vi "vision mapping.vi"(10 "GIC Input":T2={"     Use ?\nOff       On"=[FALSE, TRUE, FALSE, TRUE], "Mode:"=FALSE, "Extra Port"="", "Hokuyo Port"="COM7", "Tx Prop  Port"="COM6", "Compass Port"="", "GPS Port"="", "Num of WPs"=0, "WP Lats and Longs"={"WP Lats"=[], "WP Longs"=[]}, "Obst Lats and Longs"={"Obst Lats"=[], "Obst Longs"=[]}, "Parameters"=[], "GPS Data"=[], "Compass"=0.0, "LMS Vector"=[], "Vision Vector"=[], "Direction Cmd"=0.0, "Speed Cmd"=0.0, "WP Vector"=[], "WP Number"=0, "Extra"=0, "SW Map"=[], "Path Cluster"={"Path x node"=[], "Path y node"=[]}, "Sim Course"=[]} {"Obst Lats and Longs"."Obst Longs" format="%#_8g"; "Obst Lats and Longs"."Obst Lats" format="%#_8g"}, 11 "From vision processing":dbl[][](array[numeric])=array492x658[323736 elements]) -> (2 "GIC Output":T1={"     Use ?\nOff       On"=[FALSE, TRUE, FALSE, TRUE], "Mode:"=FALSE, "Extra Port"="", "Hokuyo Port"="COM7", "Tx Prop Port"="COM6", "Compass Port"="", "GPS Port"="", "Num of WPs"=0, "WP Lats and Longs"={"WP Lats"=[], "WP Longs"=[]}, "Obst Lats and Longs"={"Obst Lats"=[], "Obst Longs"=[]}, "Parameters"=[], "GPS Data"=[], "Compass"=0.0, "LMS Vector"=[], "Vision Vector"=[], "Direction Cmd"=0.0, "Speed Cmd"=0.0, "WP Vector"=[], "WP Number"=0, "Extra"=0, "SW Map"=[], "Path Cluster"={"Path x node"=[], "Path y node"=[]}, "Sim Course"=[]} {"Obst Lats and Longs"."Obst Longs" format="%#_8g"; "Obst Lats and Longs"."Obst Lats" format="%#_8g"})   [LabVIEW 2014]
panel:
  out "image out":T3(plugin-control)
  out "Local Map":picture
  out "tes7":dbl
  out "tes6":dbl
  out "tes5":dbl
  out "tes4":dbl
  out "tes3":dbl
  out "tes2":dbl
  out "xn2":dbl
  out "yn1":dbl
  out "xn1":dbl
  out "th":dbl
  out "ppm":dbl
  out "yp":dbl
  out "xp":dbl
  out "SwMap out":dbl[][](array[numeric])
  # "Vision Mapping"
  # "Input:"
  # "Output"
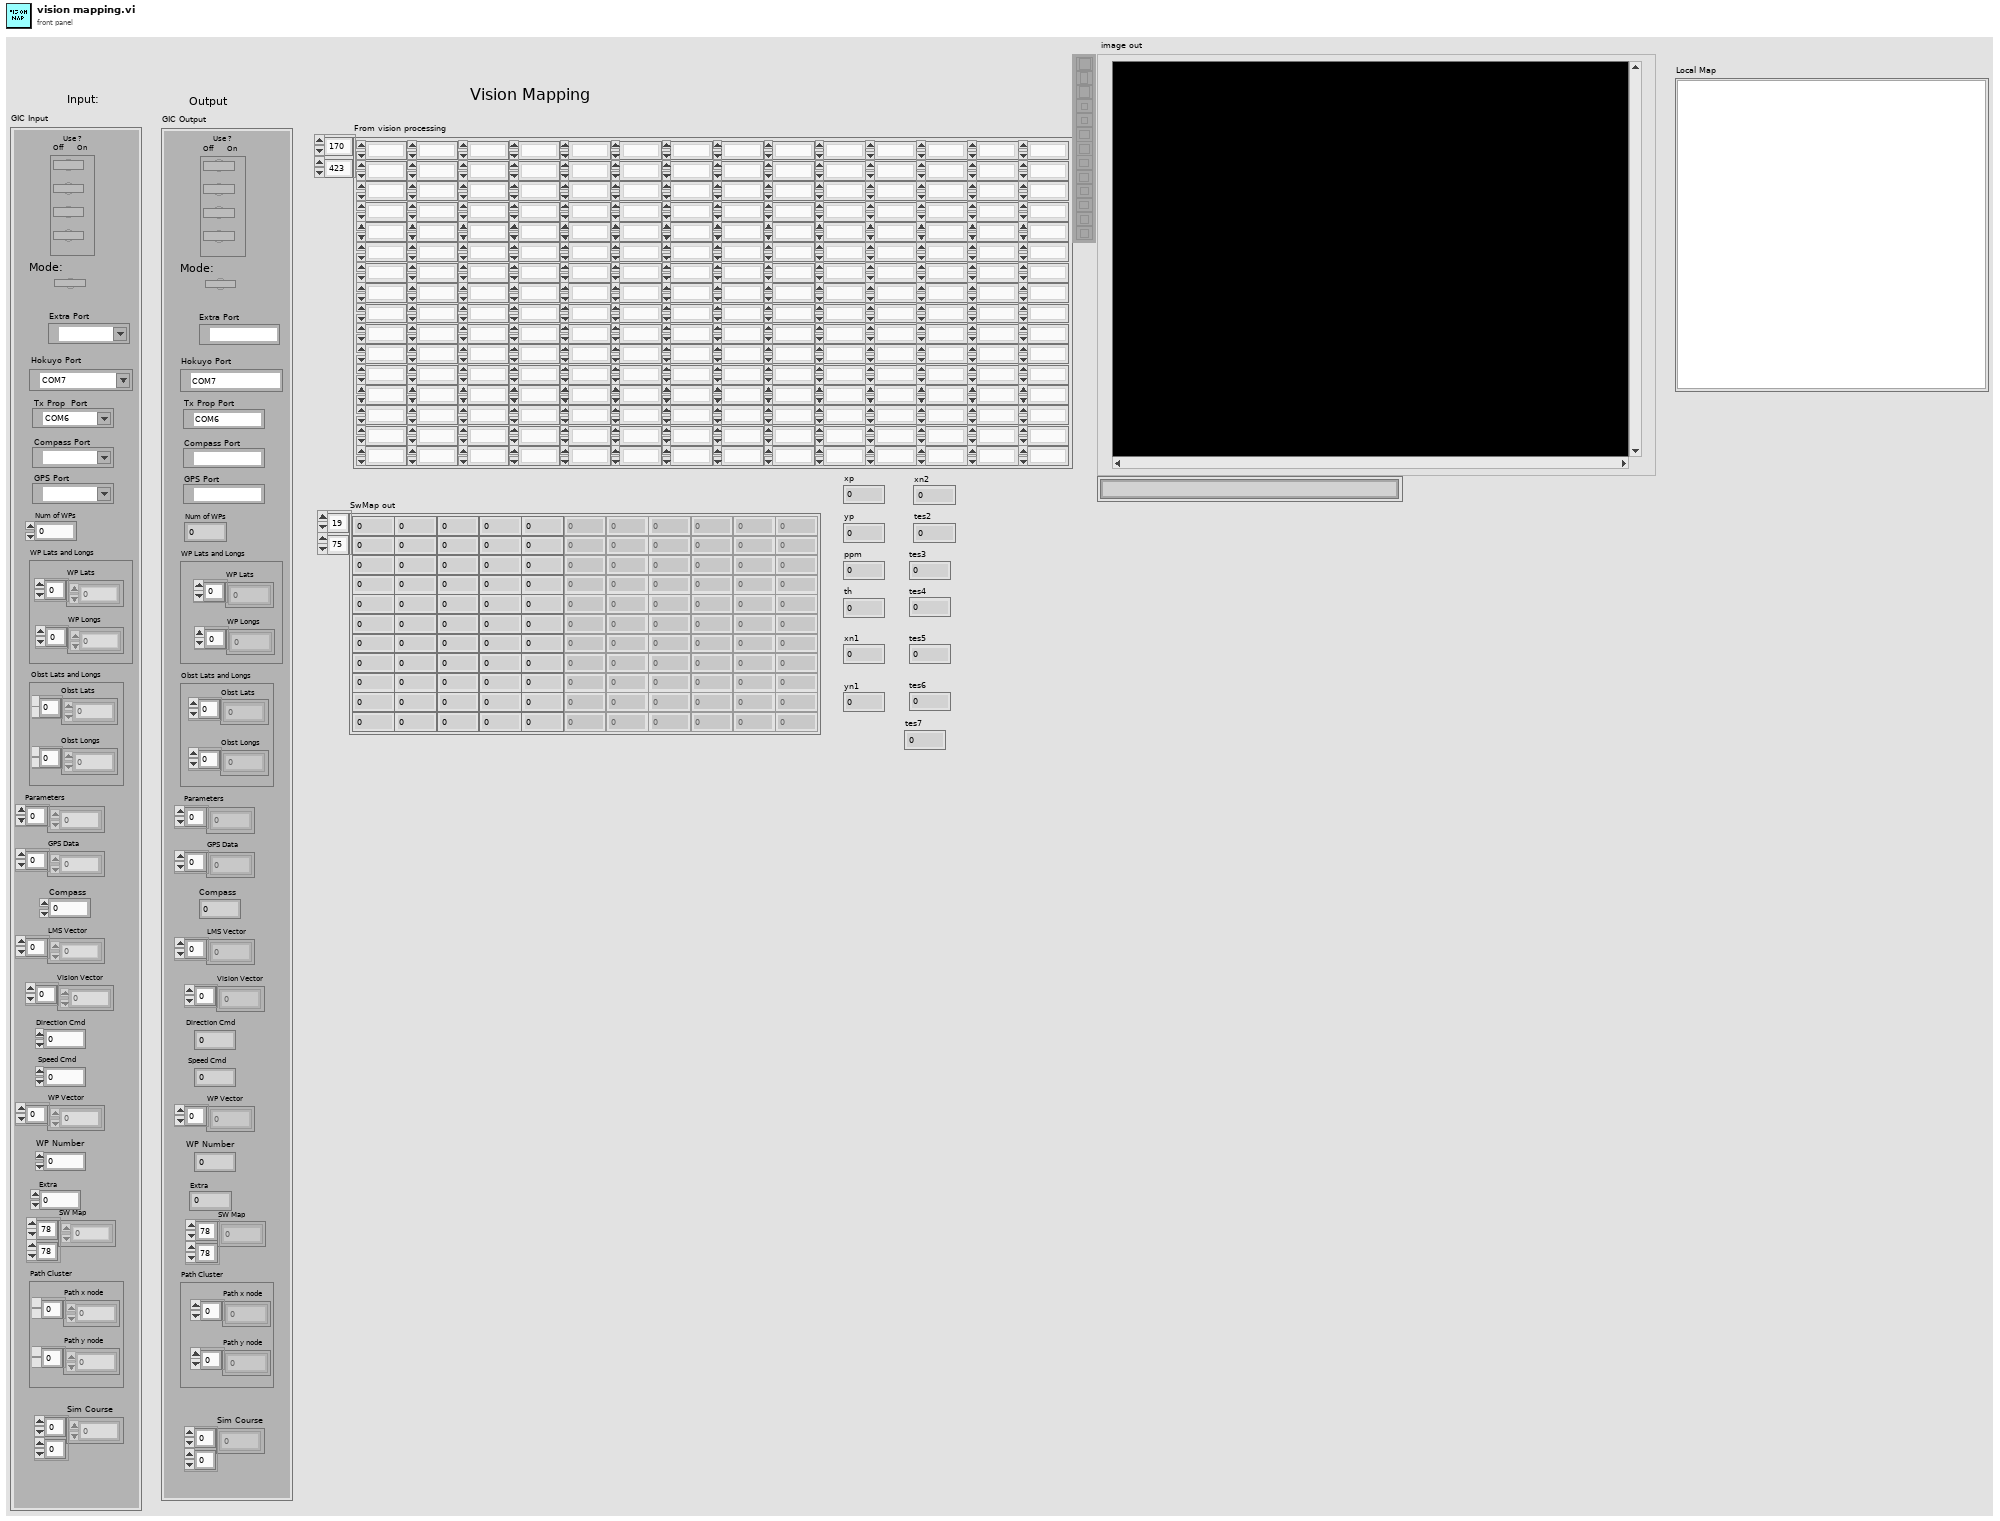
[diagram p1: front panel]
types:
  T1 = cluster{"     Use ?\nOff       On":bool[], "Mode:":bool, "Extra Port":refnum<visa-resource-name>, "Hokuyo Port":refnum<visa-resource-name>, "Tx Prop Port":refnum<visa-resource-name>, "Compass Port":refnum<visa-resource-name>, "GPS Port":refnum<visa-resource-name>, "Num of WPs":i16, "WP Lats and Longs":cluster{"WP Lats":dbl[], "WP Longs":dbl[]}, "Obst Lats and Longs":cluster{"Obst Lats":dbl[], "Obst Longs":dbl[]}, "Parameters":dbl[], "GPS Data":dbl[], "Compass":dbl, "LMS Vector":dbl[], "Vision Vector":dbl[], "Direction Cmd":dbl, "Speed Cmd":dbl, "WP Vector":dbl[], "WP Number":i32, "Extra":i16, "SW Map":i32[][], "Path Cluster":cluster{"Path x node":dbl[], "Path y node":dbl[]}, "Sim Course":i8[][]}
  T2 = cluster{"     Use ?\nOff       On":bool[], "Mode:":bool, "Extra Port":refnum<visa-resource-name>, "Hokuyo Port":refnum<visa-resource-name>, "Tx Prop  Port":refnum<visa-resource-name>, "Compass Port":refnum<visa-resource-name>, "GPS Port":refnum<visa-resource-name>, "Num of WPs":i16, "WP Lats and Longs":cluster{"WP Lats":dbl[], "WP Longs":dbl[]}, "Obst Lats and Longs":cluster{"Obst Lats":dbl[], "Obst Longs":dbl[]}, "Parameters":dbl[], "GPS Data":dbl[], "Compass":dbl, "LMS Vector":dbl[], "Vision Vector":dbl[], "Direction Cmd":dbl, "Speed Cmd":dbl, "WP Vector":dbl[], "WP Number":i32, "Extra":i16, "SW Map":i32[][], "Path Cluster":cluster{"Path x node":dbl[], "Path y node":dbl[]}, "Sim Course":i8[][]}
  T3 = typedef "IMAQ Image.ctl" = refnum<image>
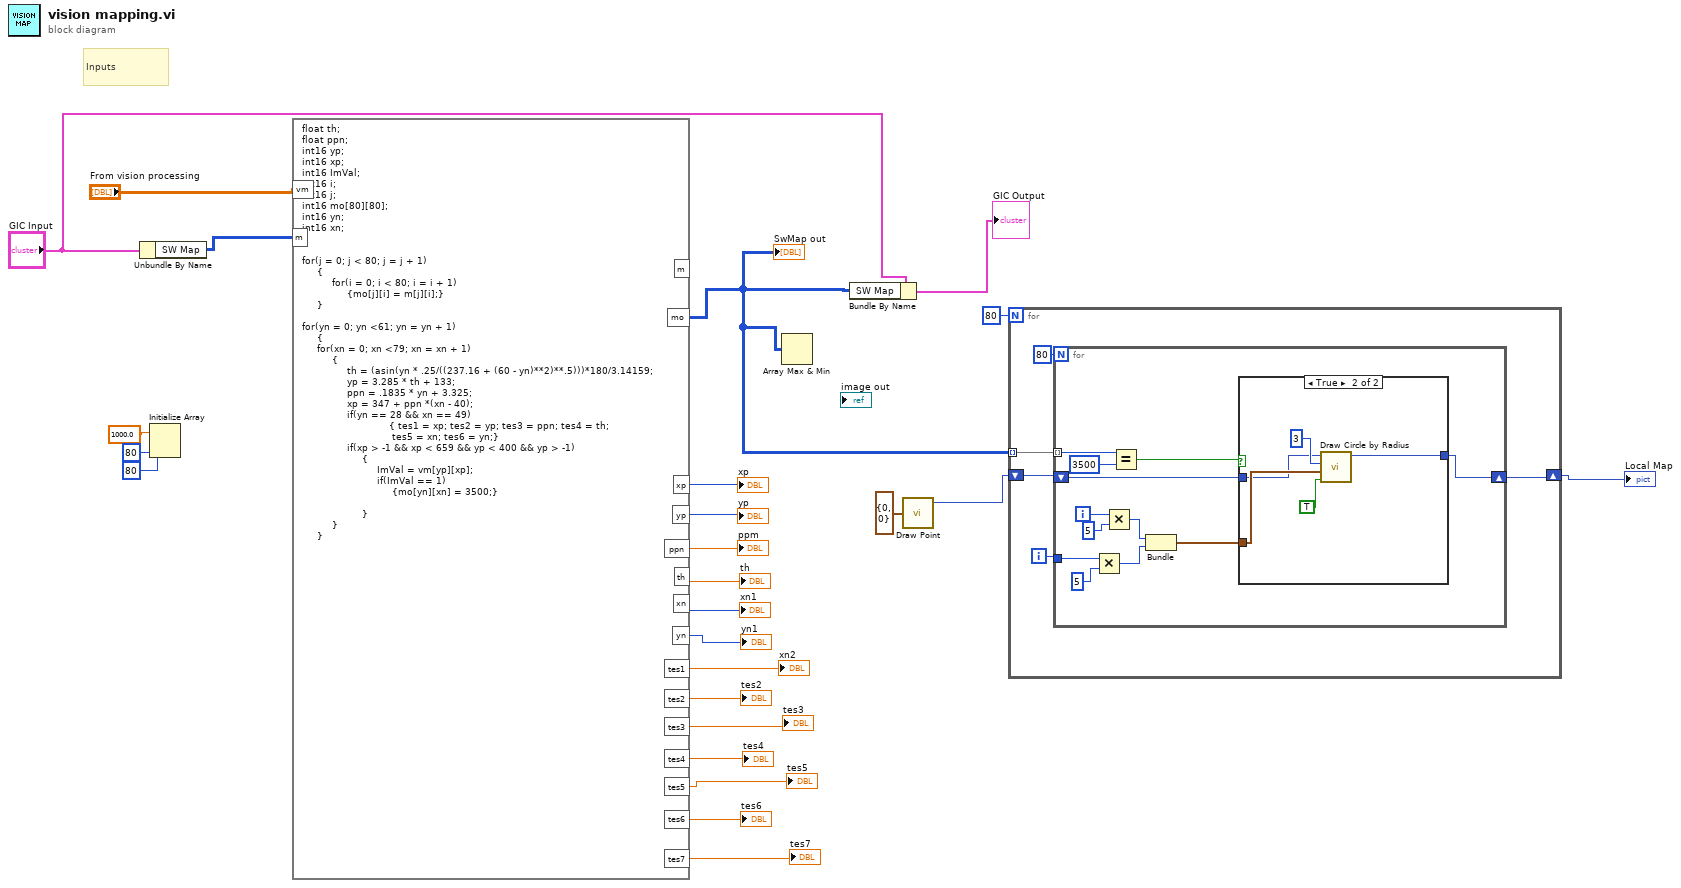
[diagram p0: block diagram]
diagram:
  # "Inputs"
  n1 = Unbundle By Name("GIC Input") -> ("SW Map"=w4:i32[][])
  n2 = Initialize Array(1000.0 ("element"), 80 ("dimension size"), 80 ("dimension size")) -> ()  [unwired: 1 out]
  n3 = formula code="float th;   \nfloat ppn;  \nint16 yp;\nint16 xp;\nint16 ImVal;\nint16 i;\nint16 j;\nint16 mo[80][80];\nint16 yn;\nint16 xn;\n\n\nfor(j = 0; j < 80; j = j + 1)\n     {\n          for(i = 0; i < 80; i = i + 1)\n               {mo[j][i] = m[j][i];}\n     }\n\nfor(yn = 0; yn <61; yn = yn + 1)\n     {\n     for(xn = 0; xn <79; xn = xn + 1)\n          {\n               th = (asin(yn * .25/((237.16 + (60 - yn)**2)**.5)))*180/3.14159;\n               yp = 3.285 * th + 133;\n               ppn = .1835 * yn + 3.325;\n               xp = 347 + ppn *(xn - 40);\n               if(yn == 28 && xn == 49)\n                             { tes1 = xp; tes2 = yp; tes3 = ppn; tes4 = th;\n                              tes5 = xn; tes6 = yn;}\n               if(xp > -1 && xp < 659 && yp < 400 && yp > -1)\n                    {\n                         ImVal = vm[yp][xp];\n                         if(ImVal == 1)\n                              {mo[yn][xn] = 3500;}\n                         \n                    }\n          }\n     }"("vm"="From vision processing", "m"=w4) -> ("mo"=w2:i16[][], "xp"=→"xp":i16, "yp"=→"yp":i16, "ppn"=→"ppm":dbl, "th"=→"th":dbl, "xn"=→"xn1":i16, "yn"=→"yn1":i16, "tes1"=→"xn2":dbl, "tes2"=→"tes2":dbl, "tes3"=→"tes3":dbl, "tes4"=→"tes4":dbl, "tes5"=→"tes5":dbl, "tes6"=→"tes6":dbl, "tes7"=→"tes7":dbl)  [unwired: 1 out]
  "SwMap out" <- w2
  n4 = Array Max & Min(array=w2) -> ()  [unwired: 4 out]
  n5 = Bundle By Name(cluster="GIC Input", "SW Map"=w2) -> (→"GIC Output":T2)
  n6 = call <vilib>:"Draw Point.vi"("point(x,y)"=cluster{"x":i16, "y":i16} {"x"=0, "y"=0}) -> ("new picture"=w6:picture)  [unwired: 8 in]
  n7 = for {
    N: 80 -> [_]
    tunnel: w2 -> [w29] mode=indexing
    shift-right: [w27] -> w7
    shift-left: w6 -> [w26]
    i -> [w28]
    n8 = for {
      N: 80 -> [_]
      tunnel: w29 -> [w42] mode=indexing
      tunnel: w28 -> [w37]
      shift-right: [w32] -> w27
      shift-left: w26 -> [w31]
      i -> [w39]
      n9 = Multiply(x=w37, y=5) -> (x*y=w34:i32)
      n10 = Multiply(x=w39, y=5) -> (x*y=w35:i32)
      n11 = Equal?(x=w42, y=i16 3500) -> (x = y?=w40:bool)
      n12 = Bundle(w35, w34) -> (w33:cluster{i32, i32})  [unwired: 1 in]
      n13 = case shown="True" w40 {
        tunnel: w33 -> [_ w46]
        tunnel: [w43 w45] -> w32
        tunnel: w31 -> [w43 w44]
        frame False {
        }
        frame True {
          n14 = call <vilib>:"Draw Circle by Radius.vi"("fill?(F)"=TRUE, "pixel center"=w46, "radius"=i16 3, "picture"=w44) -> ("new picture"=w45:picture)  [unwired: 7 in]
        }
      }
    }
  }
  "Local Map" <- w7
